vi "DID.vi"(8 "error in (no error)":errorcluster, 11 "Node Ptr":T1 format="%.0x") -> (0 "error out":errorcluster)   [LabVIEW 2013, in "Diagnostics Addon System Explorer.lvlib"]
uses:
  Diagnostics Addon System Explorer.lvlib
  <vilib>/NI Veristand/Custom Device API/Custom Device Item Ref.ctl
  Shared/FG Action.ctl
  Shared/Signal Parameters FG.vi
  Shared/GUID Lookup.vi
  <vilib>/NI Veristand/Custom Device API/NI VeriStand - Get Item Property.vi
  <vilib>/NI Veristand/Custom Device API/Get Item Property (Variant).vi
  <vilib>/NI Veristand/Custom Device API/NI VeriStand - Get Item Children.vi
  <vilib>/NI Veristand/Custom Device API/NI VeriStand - Get Custom Device Channel Data.vi
  <vilib>/NI Veristand/Custom Device API/NI VeriStand - Set Item Property.vi
  <vilib>/NI Veristand/Custom Device API/Set Item Property (Variant).vi
  <vilib>/NI Veristand/Custom Device API/Custom Device API.lvlib
  Shared/Diagnostics Addon Shared.lvlib
panel:
  in  "DID ID":u16 format="%.0x"
  out "Signals":i32(listbox)
  in  "Description":string
  in  "Name":string
  in  "SHDocVw.IWebBrowser":refnum<k7>(container)
  in  "Header":cluster{"Section Name":string}={"Section Name"="Custom Device Item Settings"}
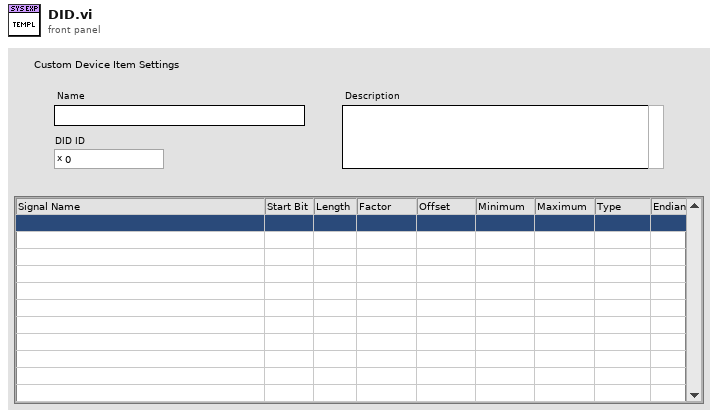
[diagram p1: front panel]
types:
  T1 = typedef "Custom Device API.lvlib/Custom Device Item Ref.ctl" = u64
  T2 = typedef "Diagnostics Addon Shared.lvlib/FG Action.ctl" = enum16{"Get", "Set"}
  T3 = typedef "Custom Device API.lvlib/Custom Device Item Info.ctl" = cluster{"Name":string, "Is Channel":bool, "GUID":string, "Is Waveform":bool}
  T4 = typedef "Diagnostics Addon Shared.lvlib/DIDPID Signal Parameters.ctl" = cluster{"Name":string, "Start Bit":u8, "Length":u8, "Scaling Factor":dbl, "Scaling Offset":dbl, "Minimum":dbl, "Maximum":dbl, "Data Type":u32, "Byte Order":u32, "Default Value":dbl, "Units":string, "Description":string}
  T5 = typedef "Custom Device API.lvlib/Custom Device Commands.ctl" = enum16{"Default", "Item renamed", "Shutdown", "Dynamic button pressed"}
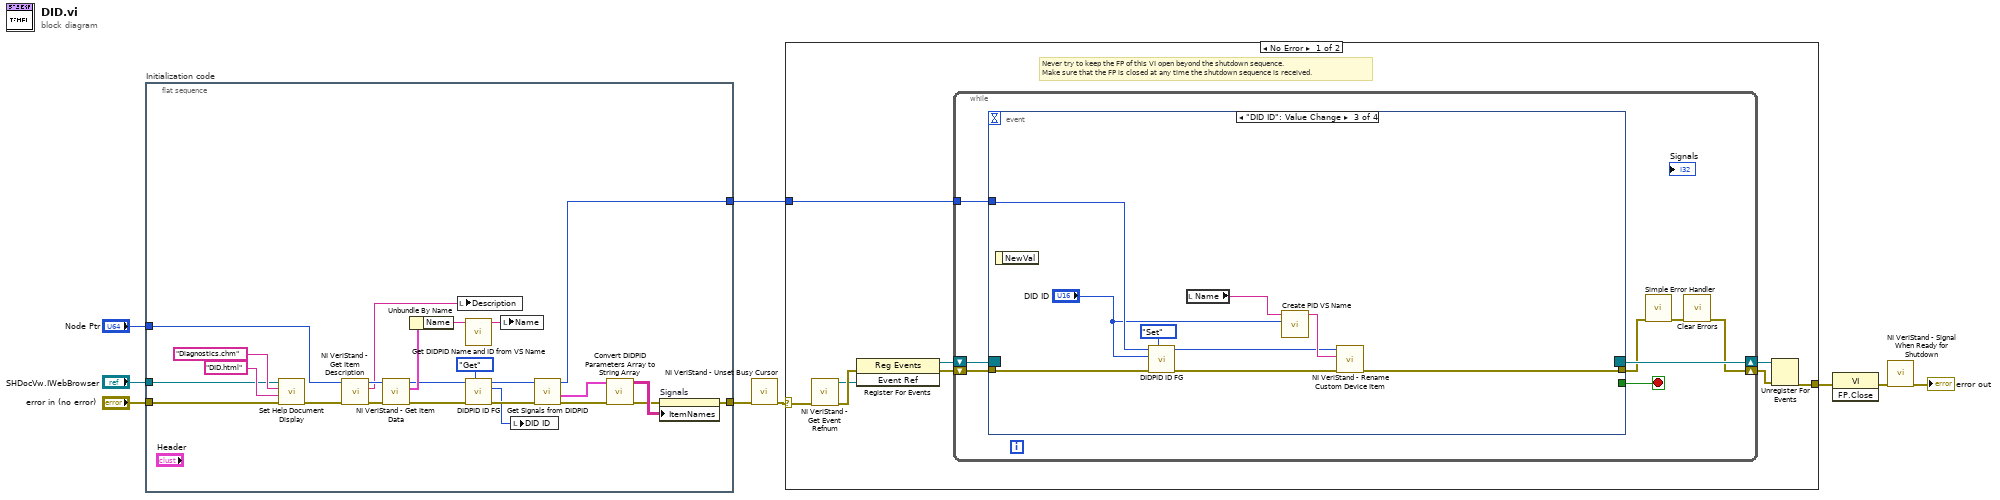
[diagram p0: block diagram]
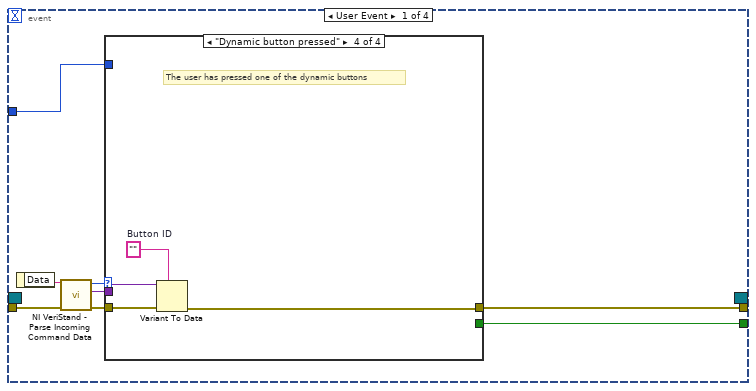
[diagram p2: hidden frame]
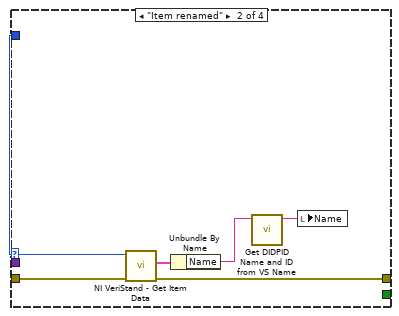
[diagram p4: hidden frame]
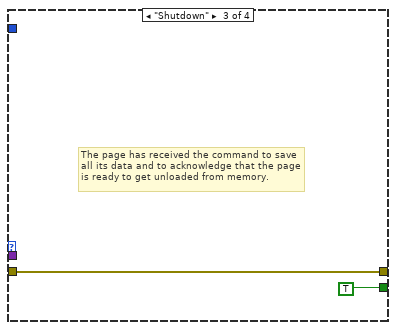
[diagram p5: hidden frame]
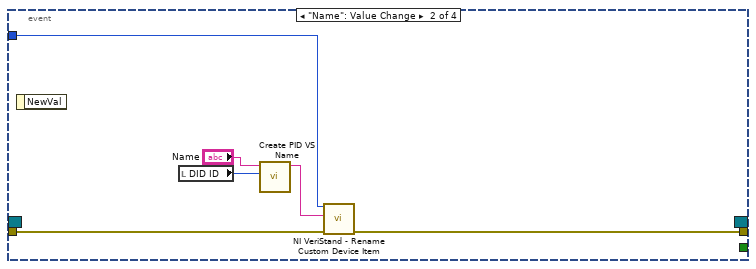
[diagram p6: hidden frame]
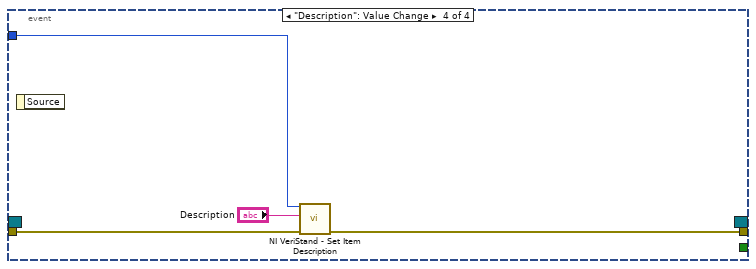
[diagram p7: hidden frame]
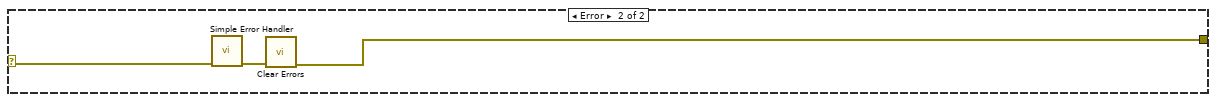
[diagram p8: hidden frame]
diagram:
  n1 = flat-sequence "Initialization code" {
    tunnel: "error in (no error)" -> [w25]
    tunnel: "Node Ptr" -> [w32]
    tunnel: [w19] -> w5
    tunnel: [w28] -> w2
    tunnel: "SHDocVw.IWebBrowser" -> [w24]
    frame #0 {
      n2 = call "Set Help Document Display.vi"("error in (no error)"=w25, "HTML File"="DID.html", "Main CHM File"="Diagnostics.chm", "SHDocVw.IWebBrowser2"=w24) -> ("error out"=w14:errorcluster)  [unwired: 7 in]
      n3 = call <vilib>:"NI VeriStand - Get Item Description.vi"("error in (no error)"=w14, "Item Ref in"=w32) -> ("error out"=w30:errorcluster, "Description"=w31:string, "Item Ref out"=w33:T1)  [unwired: 7 out]
      n4 = call <vilib>:"NI VeriStand - Get Item Data.vi"("error in (no error)"=w30, "Item Ref in"=w33) -> ("error out"=w22:errorcluster, "Item Info"=w29:T3, "Item Ref out"=w23:T1)  [unwired: 7 out]
      n5 = Unbundle By Name(w29) -> ("Name"=w12:string)
      n6 = local write "Description"(w31) -> ()
      n7 = call "Get DIDPID Name and ID from VS Name.vi"("VS PID Name"=w12) -> ("PID Name"=w11:string)  [unwired: 9 in, 1 out]
      n8 = call "DIDPID ID FG.vi"("Action"=FG_Action."Get", "error in (no error)"=w22, "Device Item Ref in"=w23) -> ("error out"=w21:errorcluster, "ID"=w13:u16, "Device Item Ref out"=w20:T1)  [unwired: 6 in]
      n9 = local write "Name"(w11) -> ()
      n10 = local write "DID ID"(w13) -> ()
      n11 = call "Get Signals from DIDPID.vi"("error in (no error)"=w21, "Device Item Ref out"=w20) -> ("error out"=w17:errorcluster, "PID Parameters"=w15:T4[], "Item Ref out"=w28:T1)  [unwired: 6 in, 1 out]
      n12 = call "Convert DIDPID Parameters Array to String Array.vi"("error in (no error)"=w17, "PID Parameters"=w15) -> ("error out"=w16:errorcluster, "PID Parameters"=w18:string[][])  [unwired: 8 in]
      n13 = property on="Signals" class="MCListbox (strict)"(error in=w16, "ItemNames"=w18) -> (error out=w19:errorcluster)  [unwired: 1 in, 1 out]
    }
  }
  n14 = call <vilib>:"NI VeriStand - Unset Busy Cursor.vi"("error in (no error)"=w5) -> ("error out"=w4:errorcluster)  [unwired: 10 out]
  n15 = case shown="No Error" w4 {
    selector: w4 -> [w34 w93]
    tunnel: [w39 w91] -> w9
    tunnel: w2 -> [w35 _]
    frame No Error {
      # "Never try to keep the FP of this VI open beyond the shutdown sequence.\nMake sure that the FP is closed at any time the shutdown sequence is received."
      n16 = call <vilib>:"NI VeriStand - Get Event Refnum.vi"("error in (no error)"=w34) -> ("error out"=w42:errorcluster, "Event Ref"=w38:refnum<user-event>)  [unwired: 9 out]
      n17 = register-events(error in=w42, w38) -> (reference out=w36:refnum<event-registration>, error out=w37:errorcluster)  [unwired: 1 in]
      n18 = while {
        tunnel: w35 -> [w46]
        shift-right: [w43] -> w40
        shift-left: w37 -> [w49]
        shift-right: [w50] -> w41
        shift-left: w36 -> [w48]
        stop <- w47 stop-if-true
        n19 = event shown="[2] \"DID ID\": Value Change" {
          selector: w48 -> [_ _ _ _]
          dyn-events: [_ _ _ _] -> w50
          timeout: _ -> [_ _ _ _]
          tunnel: w49 -> [w58 w77 w79 w89]
          tunnel: [w54 _ _ _] -> w47
          tunnel: [w53 w76 w85 w88] -> w45
          tunnel: w46 -> [w52 w75 w82 w90]
          event User Event {
            n20 = event-data() -> ("Data"=w57:string)  [unwired: 1 out]
            n21 = call <vilib>:"NI VeriStand - Parse Incoming Command Data.vi"("error in (no error)"=w58, "Incoming data"=w57) -> ("error out"=w56:errorcluster, "Outgoing data"=w51:variant, "Action"=w55:T5)  [unwired: 7 out]
            n22 = case shown="\"Dynamic button pressed\"" w55 {
              tunnel: w56 -> [w59 w65 w66 w71]
              tunnel: [_ _ TRUE _] -> w54
              tunnel: [w59 w62 w66 w68] -> w53
              tunnel: w52 -> [_ w64 _ _]
              tunnel: w51 -> [_ _ _ w70]
              frame "Default", Default {
              }
              frame "Item renamed" {
                n23 = call <vilib>:"NI VeriStand - Get Item Data.vi"("error in (no error)"=w65, "Item Ref in"=w64) -> ("error out"=w62:errorcluster, "Item Info"=w63:T3)  [unwired: 8 out]
                n24 = Unbundle By Name(w63) -> ("Name"=w61:string)
                n25 = call "Get DIDPID Name and ID from VS Name.vi"("VS PID Name"=w61) -> ("PID Name"=w60:string)  [unwired: 9 in, 1 out]
                n26 = local write "Name"(w60) -> ()
              }
              frame "Shutdown" {
                # "The page has received the command to save all its data and to acknowledge that the page is ready to get unloaded from memory."
              }
              frame "Dynamic button pressed" {
                w69 = ""  # Button ID
                # "The user has pressed one of the dynamic buttons"
                n27 = Variant To Data(error in=w71, type=w69, Variant=w70) -> (error out=w68:errorcluster)  [unwired: 1 out]
              }
            }
          }
          event "Name": Value Change {
            n28 = event-data() -> ()  [unwired: 2 out]
            n29 = local read "DID ID"() -> (w74:u16)
            n30 = call "Create PID VS Name.vi"("PID Number"=w74, "PID Name"="Name") -> ("VS Name"=w72:string)  [unwired: 9 in]
            n31 = call <vilib>:"NI VeriStand - Rename Custom Device Item.vi"("error in (no error)"=w77, "New Name"=w72, "Item Ref in"=w75) -> ("error out"=w76:errorcluster)  [unwired: 1 in, 7 out]
          }
          event "DID ID": Value Change {
            n32 = event-data() -> ()  [unwired: 2 out]
            n33 = call "DIDPID ID FG.vi"("Action"=FG_Action."Set", "error in (no error)"=w79, "ID"="DID ID", "Device Item Ref in"=w82) -> ("error out"=w78:errorcluster, "Device Item Ref out"=w81:T1)  [unwired: 5 in, 1 out]
            n34 = local read "Name"() -> (w84:string)
            n35 = call "Create PID VS Name.vi"("PID Number"="DID ID", "PID Name"=w84) -> ("VS Name"=w86:string)  [unwired: 9 in]
            n36 = call <vilib>:"NI VeriStand - Rename Custom Device Item.vi"("error in (no error)"=w78, "New Name"=w86, "Item Ref in"=w81) -> ("error out"=w85:errorcluster)  [unwired: 1 in, 7 out]
          }
          event "Description": Value Change {
            n37 = event-data() -> ()  [unwired: 2 out]
            n38 = call <vilib>:"NI VeriStand - Set Item Description.vi"("error in (no error)"=w89, "Description"="Description", "Item Ref in"=w90) -> ("error out"=w88:errorcluster)  [unwired: 8 out]
          }
        }
        n39 = call <vilib>:"Simple Error Handler.vi"("error in (no error)"=w45) -> ("error out"=w44:errorcluster)  [unwired: 1 in, 7 out]
        n40 = call <vilib>:"Clear Errors.vi"("error in (no error)"=w44) -> ("error out"=w43:errorcluster)  [unwired: 6 out]
      }
      n41 = Unregister For Events(event registration refnum=w41, error in=w40) -> (error out=w39:errorcluster)
    }
    frame Error {
      n42 = call <vilib>:"Simple Error Handler.vi"("error in (no error)"=w93) -> ("error out"=w92:errorcluster)  [unwired: 1 in, 7 out]
      n43 = call <vilib>:"Clear Errors.vi"("error in (no error)"=w92) -> ("error out"=w91:errorcluster)  [unwired: 6 out]
    }
  }
  n44 = invoke class="VI" method="FP.Close"(error in=w9) -> (error out=w8:errorcluster)  [unwired: 2 in, 2 out]
  n45 = call <vilib>:"NI VeriStand - Signal When Ready for Shutdown.vi"("error in (no error)"=w8) -> ("error out"=→"error out":errorcluster)  [unwired: 10 out]
